vi "utility_find_devices_in_project.vi"(8 "error in (no error)":errorcluster caption="错误输入（无错误）") -> (0 "error out":errorcluster caption="错误输出")   [LabVIEW 2015]
panel:
  in  "device tree in project":string(tree) caption="项目中的设备树"
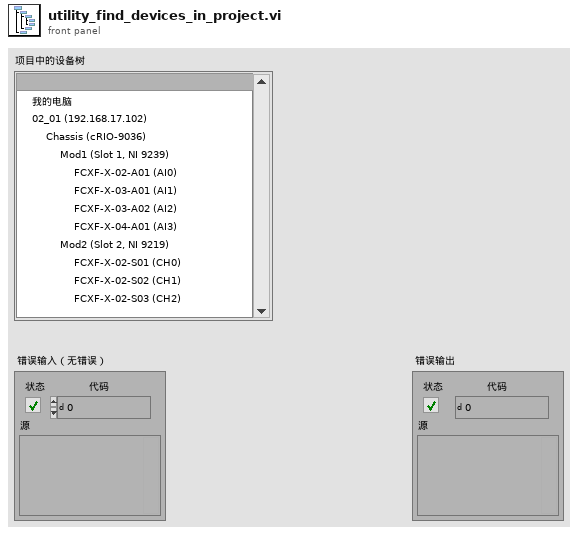
[diagram p1: front panel]
types:
  T1 = enum32{"None", "LabVIEW", "Mac OS", "Windows", "Default"}
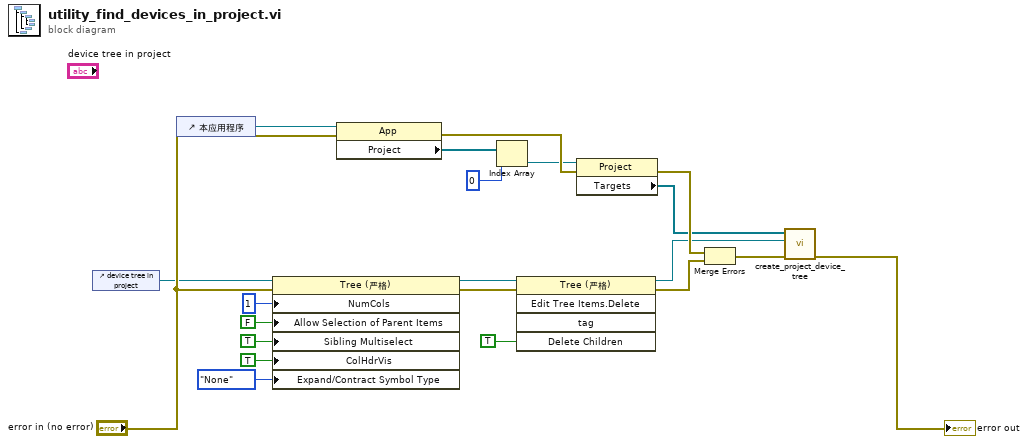
[diagram p0: block diagram]
diagram:
  n1 = control-ref of="device tree in project"() -> (w1:refnum<vi>)
  n2 = control-ref of="本应用程序"() -> (w16:refnum<vi>)
  n3 = property class="Tree (严格)"(reference=w1, error in="error in (no error)", "NumCols"=u32 1 ("列数"), "Allow Selection of Parent Items"=FALSE ("允许选择父项"), "Sibling Multiselect"=TRUE ("同辈多选"), "ColHdrVis"=TRUE ("允许选择父项"), "Expand/Contract Symbol Type"=T1."None" ("缩进/移出符号:符号类型")) -> (reference out=w12:refnum<vi>, error out=w11:errorcluster)
  n4 = property class="App"(reference=w16, error in="error in (no error)") -> (error out=w19:errorcluster, "Project"=w20:refnum<vi>[])  [unwired: 1 out]
  n5 = Index Array(array=w20, index=0 ("索引")) -> (element=w18:refnum<vi>)
  n6 = invoke class="Tree (严格)" method="Edit Tree Items.Delete"(reference=w12, error in=w11, "Delete Children"=TRUE ("删除子项？")) -> (reference out=w2:refnum<vi>, error out=w7:errorcluster)  [unwired: 2 in, 3 out]
  n7 = property class="Project"(reference=w18, error in=w19) -> (error out=w4:errorcluster, "Targets"=w3:refnum<vi>[])  [unwired: 1 out]
  n8 = Merge Errors(w4, w7) -> (w5:errorcluster)
  n9 = call "create_project_device_tree.vi"("error in (no error)"=w5, "Tree Control Ref"=w2, "Project Item Array"=w3) -> ("error out"=→"error out":errorcluster)  [unwired: 8 in]
